vi "HW_Linearise_+_temp_comp.vi"(5 "Caib const":dbl[](array[numeric]) format="%.4f", 6 "HW voltage":dbl[](array[numeric]) format="%.4f") -> (0 "Velocity":dbl[](array[numeric]) format="%.2f")   [LabVIEW 2010]
uses:
  Globals/Meas_global.vi
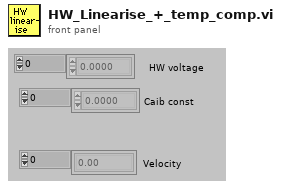
[diagram p1: front panel]
types:
  T1 = cluster{"Caib const[0]":dbl, "Caib const[1]":dbl, "Caib const[2]":dbl, "Caib const[3]":dbl, "Caib const[4]":dbl, "Caib const[5]":dbl, "Caib const[6]":dbl, "Caib const[7]":dbl}
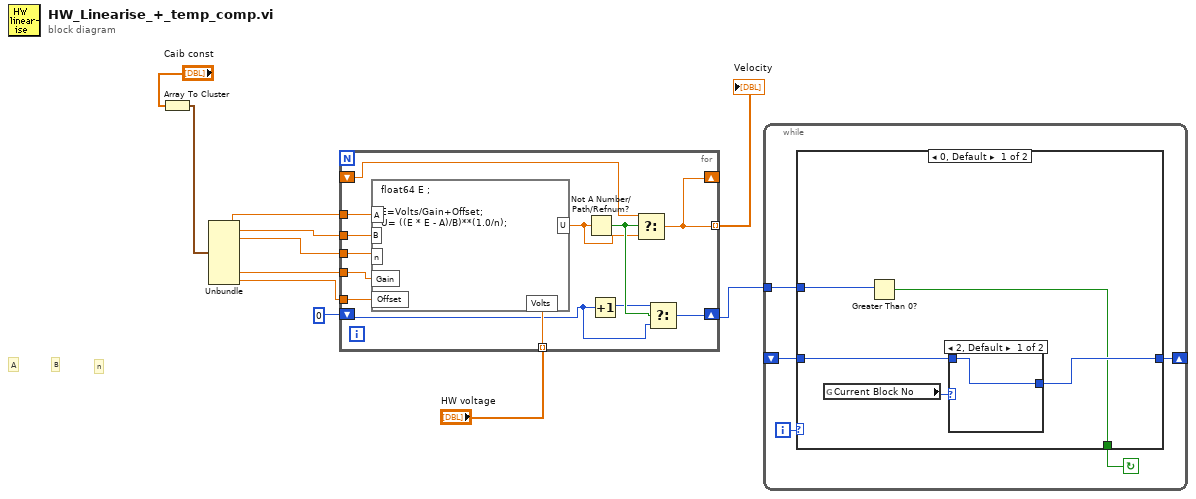
[diagram p0: block diagram]
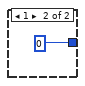
[diagram p2: hidden frame]
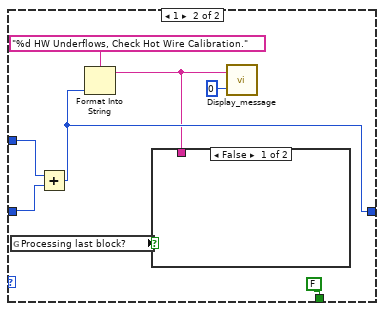
[diagram p3: hidden frame]
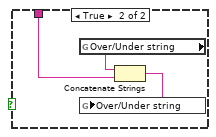
[diagram p4: hidden frame]
diagram:
  # "n"
  # "B"
  # "A"
  n1 = Array To Cluster(array="Caib const") -> (cluster=w9:T1)
  n2 = Unbundle(w9) -> ("Caib const[0]"=w8:dbl, "Caib const[1]"=w7:dbl, "Caib const[2]"=w6:dbl, "Caib const[6]"=w2:dbl, "Caib const[7]"=w1:dbl)  [unwired: 3 out]
  n3 = for {
    tunnel: "HW voltage" -> [w24] mode=indexing
    tunnel: w8 -> [w23]
    tunnel: w7 -> [w22]
    tunnel: w6 -> [w21]
    shift-right: [w14] -> _
    shift-left: _ -> [w20]
    tunnel: [w14] -> w5 mode=indexing
    shift-right: [w16] -> w3
    shift-left: 0 -> [w18]
    tunnel: w2 -> [w13]
    tunnel: w1 -> [w12]
    n4 = formula code="float64 E ;\n\nE=Volts/Gain+Offset;\nU= ((E * E - A)/B)**(1.0/n);"("A"=w23, "n"=w21, "B"=w22, "Volts"=w24, "Gain"=w13, "Offset"=w12) -> ("U"=w15:dbl)
    n5 = Not A Number/Path/Refnum?(number/path/refnum=w15) -> (NaN/Path/Refnum?=w19:bool)
    n6 = Increment(x=w18) -> (x+1=w17:i32)
    n7 = Select(t=w20, s=w19, f=w15) -> (s? t:f=w14:dbl)
    n8 = Select(t=w17, s=w19, f=w18) -> (s? t:f=w16:i32)
  }
  "Velocity" <- w5
  n9 = while {
    shift-left: _ -> [w26]
    shift-right: [w27] -> _
    tunnel: w3 -> [w29]
    i -> [w25]
    stop <- w28 continue-if-true
    n10 = case shown="0, Default" w25 {
      tunnel: w29 -> [w31 w37]
      tunnel: [w30 FALSE] -> w28
      tunnel: [w33 w39] -> w27
      tunnel: w26 -> [w32 w42]
      frame 0, Default {
        n11 = global read "Meas_global.vi" "Current Block No"() -> (w34:i32)
        n12 = Greater Than 0?(x=w31) -> (x > 0?=w30:bool)
        n13 = case shown="2, Default" w34 {
          tunnel: [w35 0] -> w33
          tunnel: w32 -> [w35 _]
          frame 2, Default {
          }
          frame 1 {
          }
        }
      }
      frame 1 {
        n14 = global read "Meas_global.vi" "Processing last block?"() -> (w40:bool)
        n15 = Add(x=w37, y=w42) -> (x+y=w39:i32)
        n16 = Format Into String(format string="%d HW Underflows, Check Hot Wire Calibration." ("Format String"), w39) -> (resulting string=w38:string)  [unwired: 2 in, 1 out]
        n17 = case shown="False" w40 {
          tunnel: w38 -> [_ w45]
          frame False {
          }
          frame True {
            n18 = global read "Meas_global.vi" "Over/Under string"() -> (w47:string)
            n19 = Concatenate Strings(w47, w45) -> (w46:string)
            n20 = global write "Meas_global.vi" "Over/Under string"(w46) -> ()
          }
        }
        n21 = call "Display_message.vi"("Time to display message"=u32 0, "Message"=w38) -> ()  [unwired: 2 out]
      }
    }
  }
